vi "Test.vi"() -> ()   [LabVIEW 2025, in "PID.lvlib" / "PID.lvclass"]
uses:
  PID/PID.lvclass
  PID/PID.lvclass/PID.ctl
  <vilib>/ptbypt/NI_PtbyPt.lvlib
panel:
  out "Error":cluster{"Current":dbl, "Previous":dbl}
  in  "PID Gains":cluster{"Kp":dbl, "Ki":dbl, "Kd":dbl}
  out "Waveform Chart 2":dbl(graph)
  out "Waveform Chart":dbl(graph)
  in  "Setpoint":dbl
  in  "stop":bool
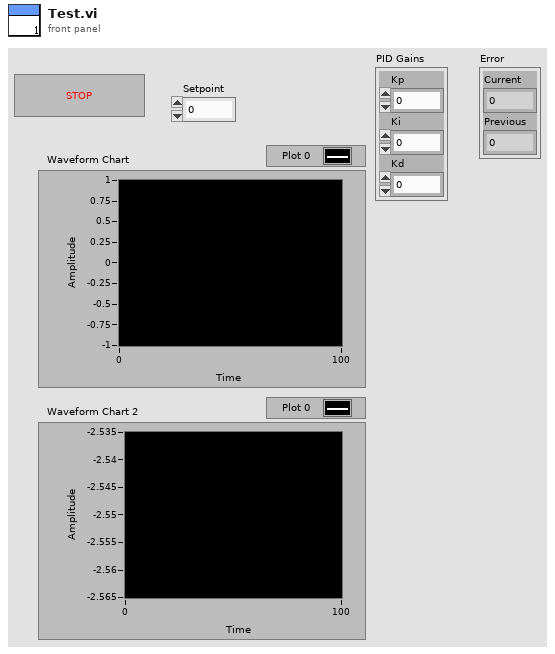
[diagram p1: front panel]
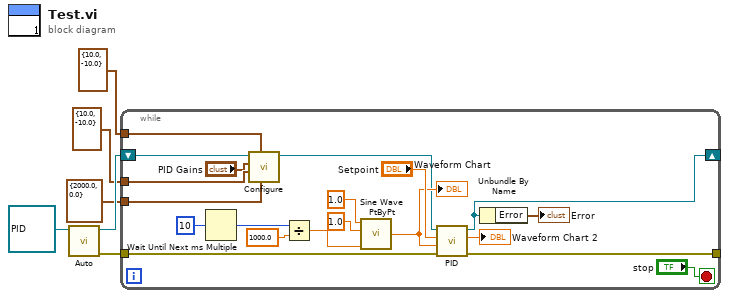
[diagram p0: block diagram]
diagram:
  n1 = call-dynamic "Auto.vi"("PID in"=refnum<class "PID.lvclass"> refnum) -> ("error out"=w6:errorcluster, "PID out"=w5:refnum<class "PID.lvclass">)  [unwired: 9 in]
  n2 = while {
    shift-right: [w8] -> _
    shift-left: w5 -> [w11]
    tunnel: w6 -> [w25]
    tunnel: [w24] -> _
    tunnel: cluster{"Max":dbl, "Min":dbl} {"Max"=2000.0, "Min"=0.0} ("Setpoint Range") -> [w14]
    tunnel: cluster{"Max":dbl, "Min":dbl} {"Max"=10.0, "Min"=-10.0} ("Process Span") -> [w13]
    tunnel: cluster{"Max":dbl, "Min":dbl} {"Max"=10.0, "Min"=-10.0} ("Output Range") -> [w12]
    stop <- "stop" stop-if-true
    n3 = Wait Until Next ms Multiple(millisecond multiple=u32 10) -> (millisecond timer value=w19:u32)
    n4 = call-dynamic "Configure.vi"("Setpoint Range"=w14, "Process Span"=w13, "Output Range"=w12, "PID Gains"="PID Gains", "PID in"=w11) -> ("PID out"=w10:refnum<class "PID.lvclass">)  [unwired: 5 in, 1 out]
    n5 = Divide(x=w19, y=1000.0) -> (x/y=w17:dbl)
    n6 = call <vilib>:"Sine Wave PtByPt.vi"("time"=w17, "frequency"=1.0, "amplitude"=1.0) -> ("sine wave"=w16:dbl)  [unwired: 1 in]
    "Waveform Chart" <- w16
    n7 = call-dynamic "PID.vi"("error in (no error)"=w25, "Process Variable"=w16, "Setpoint"="Setpoint", "PID in"=w10) -> ("error out"=w24:errorcluster, "Output"=→"Waveform Chart 2":dbl, "PID out"=w8:refnum<class "PID.lvclass">)  [unwired: 5 in]
    n8 = Unbundle By Name(w8) -> ("Error"=→"Error":cluster{"Current":dbl, "Previous":dbl})
  }
